vi "SDSU_GetClks.vi"(10 "DACS":string[][](table)) -> (2 "Table":string[][](table))   [LabVIEW 2016]
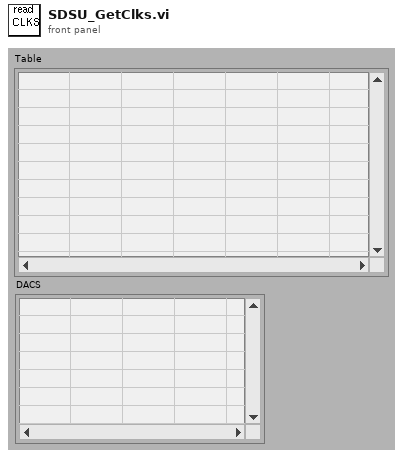
[diagram p1: front panel]
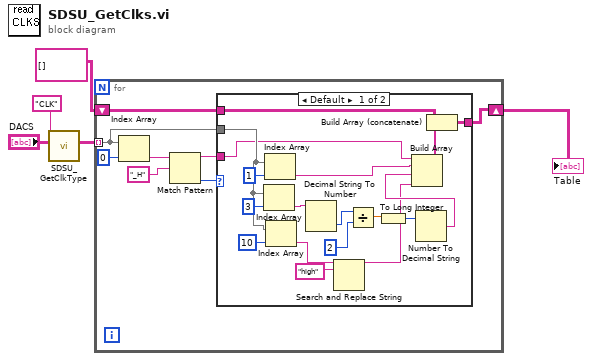
[diagram p0: block diagram]
diagram:
  n1 = call "SDSU_GetClkType.vi"("TableIn"="DACS", "type"="CLK") -> ("Table Out"=w4:string[][])  [unwired: 9 out]
  n2 = for {
    tunnel: w4 -> [w9] mode=indexing
    shift-right: [w7] -> w3
    shift-left: string[][] [] -> [w6]
    n3 = Index Array(array=w9, index=0) -> (element=w12:string)
    n4 = Match Pattern(string=w12, regular expression="_H") -> (before substring=w8:string, offset past match=w10:i32)  [unwired: 3 out]
    n5 = case shown="Default" w10 {
      tunnel: w9 -> [w29 _]
      tunnel: w8 -> [w23 _]
      tunnel: [w19 w32] -> w7
      tunnel: w6 -> [w18 w32]
      frame Default {
        n6 = Index Array(array=w29, index=3) -> (element=w28:string)
        n7 = Index Array(array=w29, index=1) -> (element=w22:string)
        n8 = Index Array(array=w29, index=10) -> (element=w16:string)
        n9 = Decimal String To Number(string=w28) -> (number=w27:i32)  [unwired: 3 out]
        n10 = Search and Replace String(input string=w16, search string="high") -> (result string=w14:string)  [unwired: 1 in, 8 out]
        n11 = Divide(x=w27, y=2) -> (x/y=w25:dbl)
        n12 = To Long Integer(number=w25) -> (32bit integer=w24:i32)
        n13 = Number To Decimal String(number=w24) -> (decimal integer string=w21:string)  [unwired: 1 out]
        n14 = Build Array(w23, w22, w21, w14) -> (w20:string[])
        n15 = Build Array (concatenate)(w18, w20) -> (w19:string[][])
      }
      frame -1 {
      }
    }
  }
  "Table" <- w3
